vi "Periodic Tasks.vi"(8 "error in":errorcluster) -> ()   [LabVIEW 2020]
doc: "This VI runs in parallel to other tasks. It can contain as many user-defined periodic loops as you need. These can carry out PID or other sorts of timed response."
uses:
  <vilib>/Rock Robotics/WPI/ThirdParty/REV Robotics/REVLib/Typedef/Spark MAX Control Type.ctl
  <vilib>/Rock Robotics/WPI/Utilities/WPI_GetSetVariantRefNum.vi
panel:
  in  "Right Setpoint":dbl
  out "Right PID Chart":T1(graph)
  in  "Right PID Constants":T2={"P Gain"=0.0, "I Gain"=0.0, "D Gain"=0.0, "F Gain"=0.0, "I Zone"=0.0, "Min Output"=-1.0, "Max Output"=1.0} {"Max Output" min=-1.0 max=1.0 step=0.01; "Min Output" min=-1.0 max=1.0 step=0.01; "I Zone" step=0.01; "F Gain" step=0.01; "D Gain" step=0.01; "I Gain" step=0.01; "P Gain" min=0.0 step=0.01}
  in  "Left Setpoint":dbl
  out "Left PID Chart":T1(graph)
  in  "Left PID Constants":T2={"P Gain"=0.0, "I Gain"=0.0, "D Gain"=0.0, "F Gain"=0.0, "I Zone"=0.0, "Min Output"=-1.0, "Max Output"=1.0} {"Max Output" min=-1.0 max=1.0 step=0.01; "Min Output" min=-1.0 max=1.0 step=0.01; "I Zone" step=0.01; "F Gain" step=0.01; "D Gain" step=0.01; "I Gain" step=0.01; "P Gain" min=0.0 step=0.01}
  # "Click here to set max"
  # "Click here to set min"
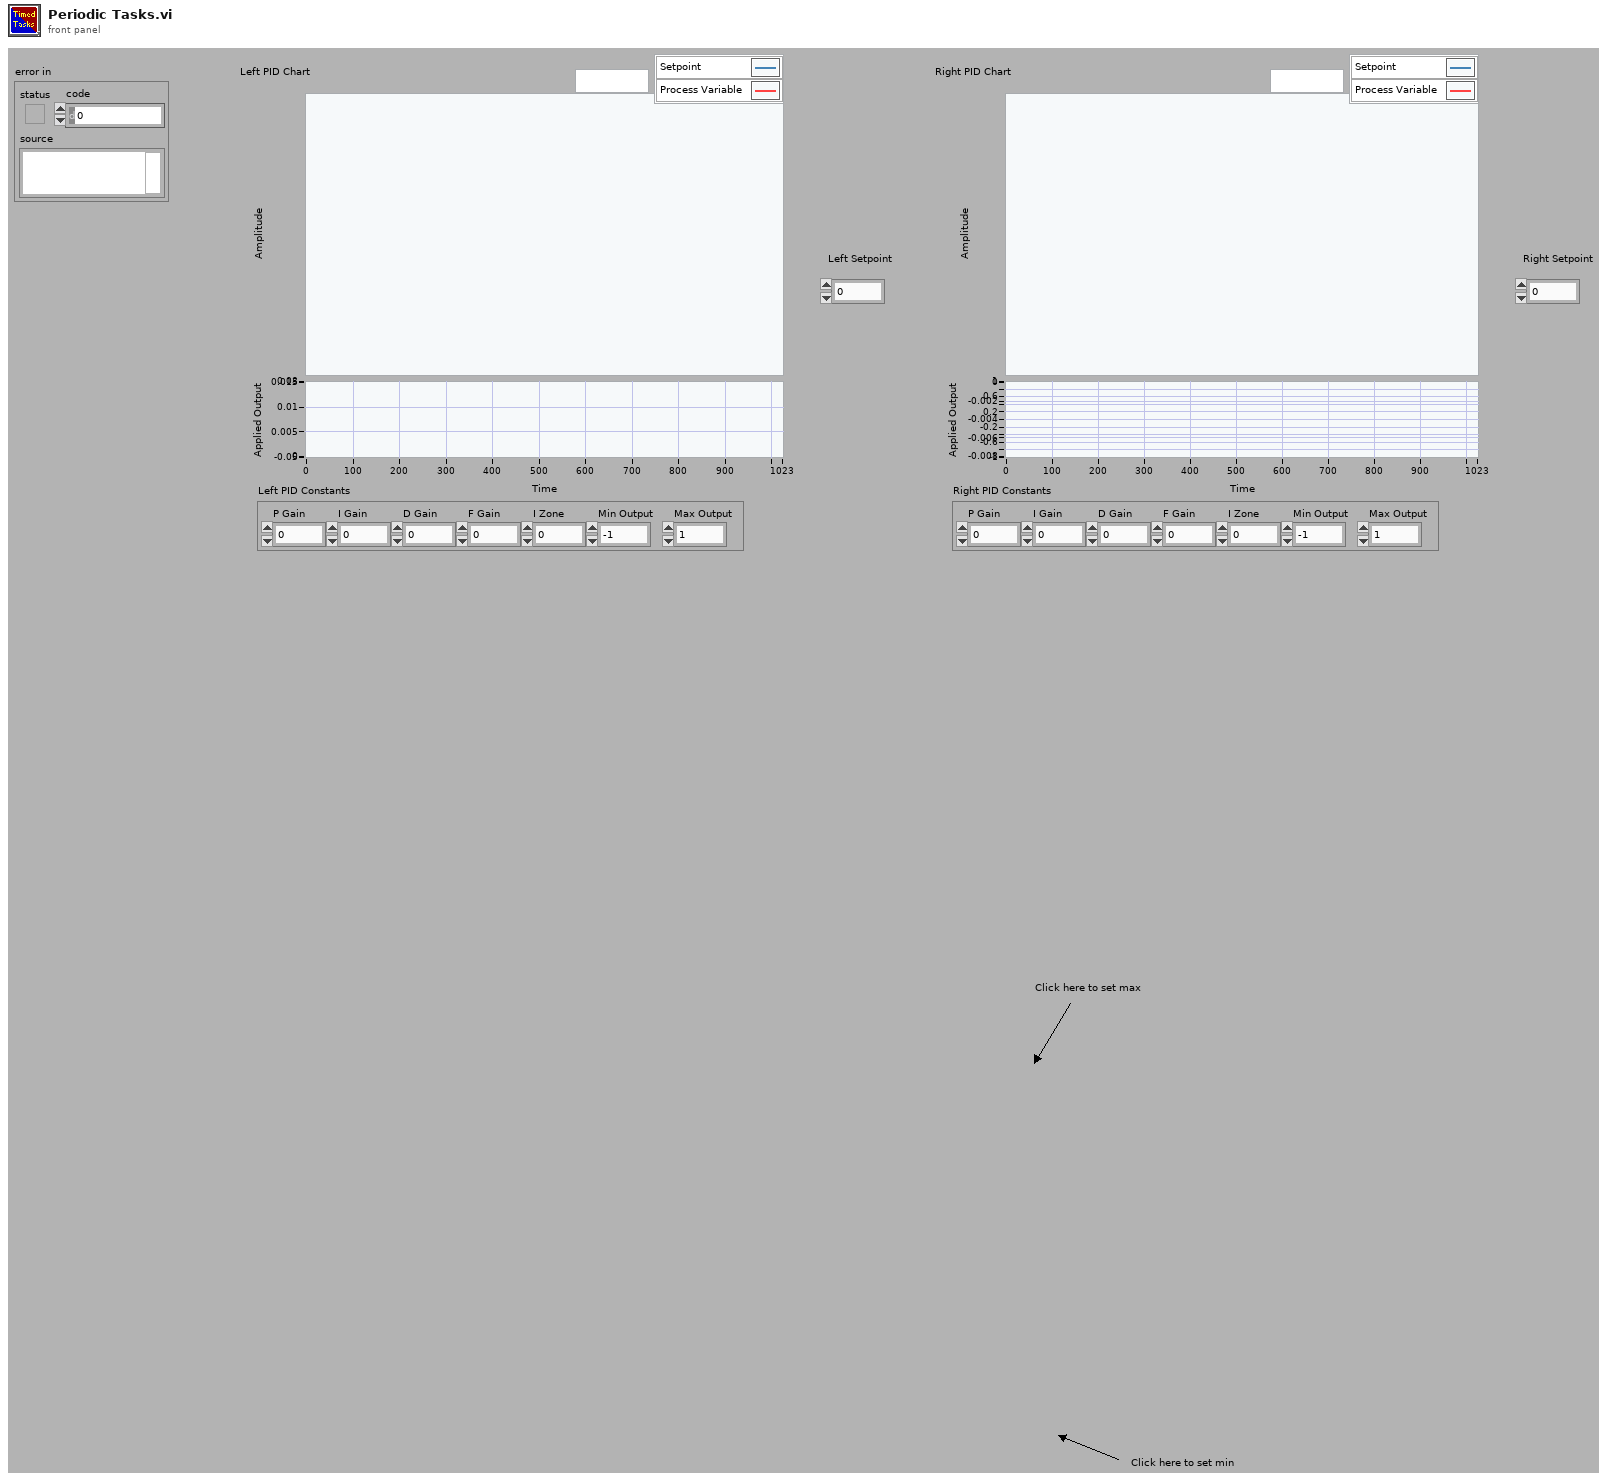
[diagram p1: front panel]
types:
  T1 = cluster{"Sensor Velocity":dbl, "Setpoint":dbl, "Applied Output":dbl}
  T2 = cluster{"P Gain":dbl, "I Gain":dbl, "D Gain":dbl, "F Gain":dbl, "I Zone":dbl, "Min Output":dbl, "Max Output":dbl}
  T3 = typedef "WPI_JoystickDevRef.ctl" = cluster{"Device":T4}
  T4 = typedef "WPI_JoystickDeviceEnum.ctl" = enum16{"USB 0", "USB 1", "USB 2", "USB 3", "USB 4", "USB 5"}
  T5 = typedef "WPI_RobotDriveDevRef.ctl" = cluster{"DevStatus":errorcluster, "Motors[]":T6[], "Square Inputs":bool, "Max Output":dbl}
  T6 = typedef "WPI_MotorControlDeviceRef.ctl" = cluster{"DeviceStatus":errorcluster, "Type":T7, "PWM":cluster{"PWM Channel":T8, "DeadBand":T9}, "CAN":cluster{"Device Number":u8, "SetOutput VI Ref":variant, "GetOutput VI Ref":variant, "Enable VI Ref":variant, "Disable VI Ref":variant, "Data":variant}, "Invert":bool, "DIO PWM":cluster{"PWM \"Enable\" Channel":T8, "DIOChannel":T10, "PWM Rate":dbl}}
  T7 = typedef "WPI_MotorControlType.ctl" = enum16{"PWM", "CAN", "DIO PWM"}
  T8 = typedef "FPGA_DIOPWMChannel.ctl" = enum8{"PWM 0", "PWM 1", "PWM 2", "PWM 3", "PWM 4", "PWM 5", "PWM 6", "PWM 7", "PWM 8", "PWM 9", "PWM MXP 0", "PWM MXP 1", "PWM MXP 2", "PWM MXP 3", "PWM MXP 4", "PWM MXP 5", "PWM MXP 6", "PWM MXP 7", "PWM MXP 8", "PWM MXP 9", "Invalid"}
  T9 = typedef "WPI_PWMDeadband.ctl" = cluster{"Name":string, "maxPositivePwm":i32, "minPositivePwm":i32, "centerPwm":i32, "maxNegativePwm":i32, "minNegativePwm":i32, "angularRange":u16}
  T10 = typedef "FPGA_DIOChannel.ctl" = enum8{"DIO 0", "DIO 1", "DIO 2", "DIO 3", "DIO 4", "DIO 5", "DIO 6", "DIO 7", "DIO 8", "DIO 9", "DIO MXP 0", "DIO MXP 1", "DIO MXP 2", "DIO MXP 3", "DIO MXP 4", "DIO MXP 5", "DIO MXP 6", "DIO MXP 7", "DIO MXP 8", "DIO MXP 9", "DIO MXP 10", "DIO MXP 11", "DIO MXP 12", "DIO MXP 13", "DIO MXP 14", "DIO MXP 15", "SPI Port CS1", "SPI Port CS2", "SPI Port CS3", "SPI Port MISO", "SPI Port MOSI", "Invalid"}
  T11 = cluster{"JoystickDevRef":T3, "RobotDriveDevRef":T5}
  T12 = typedef "Spark MAX Control Type.ctl" = enum16{"Percent VBus", "Voltage", "Velocity", "Position", "Smart Motion", "Current", "Smart Velocity"}
  T13 = cluster{"P Gain":bool, "I Gain":bool, "D Gain":bool, "F Gain":bool, "I Zone":bool, "Min Output":bool, "Max Output":bool}
  T14 = typedef "Spark MAX Status 2 Frame.ctl" = cluster{"Sensor Position":dbl, "IAccum":dbl, "Timestamp":u32}
  T15 = typedef "Spark MAX Status 0 Frame.ctl" = cluster{"Applied Output":dbl, "Faults":T16, "Sticky Faults":T16, "Rsvd":u8, "Status 0 Flags":T17, "Timestamp":u32}
  T16 = typedef "Spark MAX Faults.ctl" = cluster{"Hard Limit Rev":bool, "Hard Limit Fwd":bool, "Soft Limit Fwd":bool, "Soft Limit Rev":bool, "Other Fault":bool, "DRV Fault":bool, "Has Reset?":bool, "CAN RX":bool, "CAN TX":bool, "EEPROM CRC":bool, "Stall":bool, "Sensor Fault":bool, "Motor Type Fault":bool, "IWDT Reset":bool, "Over Current":bool, "Brownout":bool}
  T17 = typedef "Spark MAX Status 0 Flags.ctl" = cluster{"Invert/Brake":bool, "Is Follower":bool}
  T18 = cluster{"Sensor Position":dbl, "Right Setpoint":dbl, "Applied Output":dbl}
  T19 = cluster{"Sensor Position":dbl, "Left Setpoint":dbl, "Applied Output":dbl}
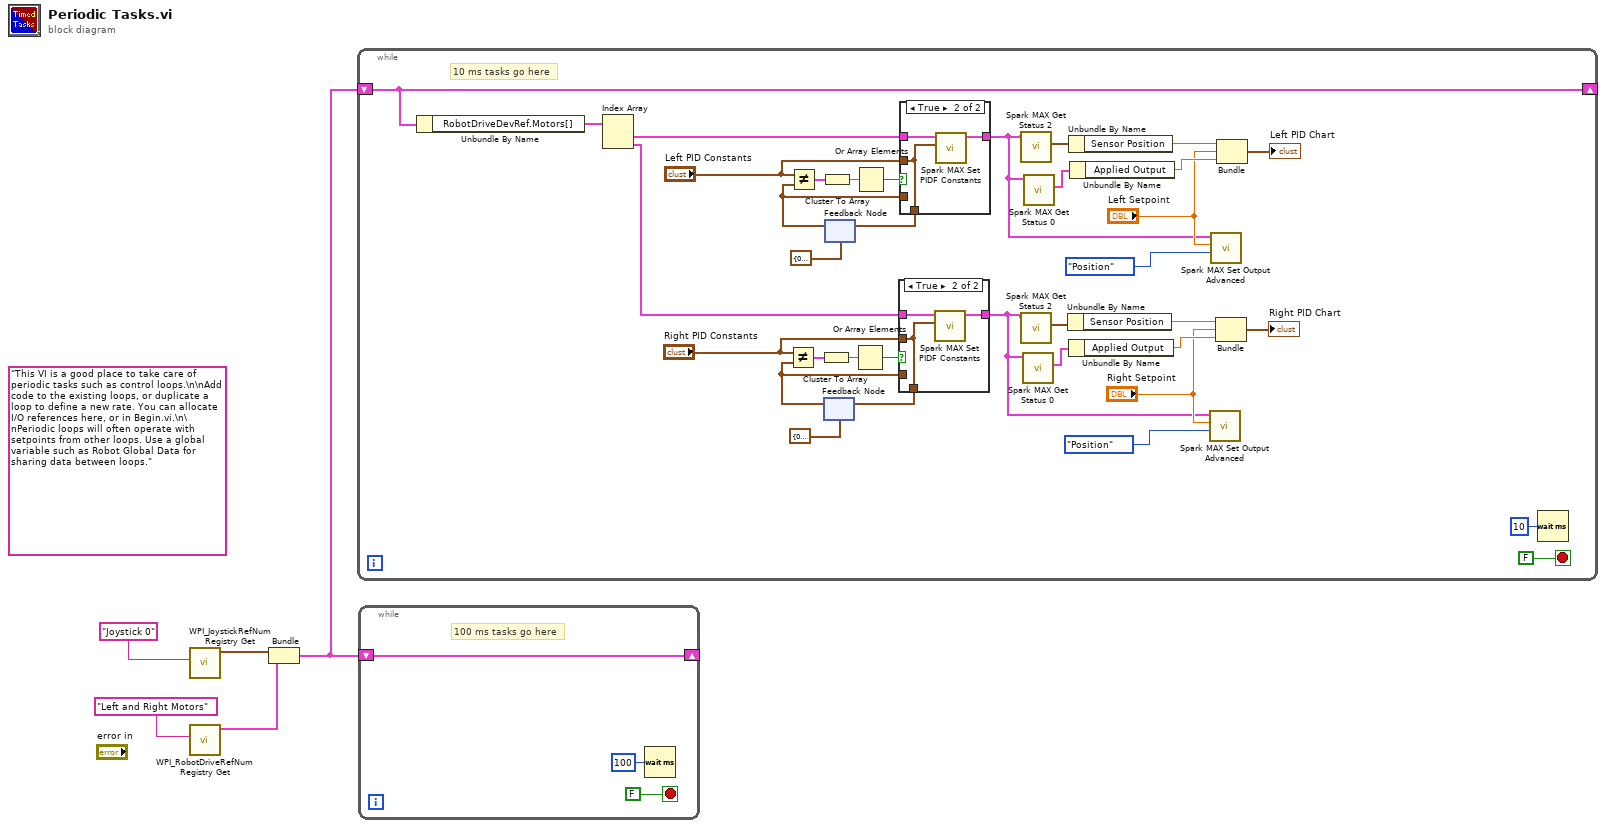
[diagram p0: block diagram]
diagram:
  (unwired) "This VI is a good place to take care of periodic tasks such as control loops.\n\nAdd code to the existing loops, or duplicate a loop to define a new rate. You can allocate I/O references here, or in Begin.vi.\n\nPeriodic loops will often operate with setpoints from other loops. Use a global variable such as Robot Global Data for sharing data between loops."
  n1 = call <vilib>:"WPI_JoystickRefNum Registry Get.vi"("refnum name"="Joystick 0") -> ("JoystickDevRef"=w3:T3)  [unwired: 1 in, 9 out]
  n2 = call <vilib>:"WPI_RobotDriveRefNum Registry Get.vi"("refnum name"="Left and Right Motors") -> ("RobotDriveDevRef"=w2:T5)  [unwired: 1 in, 9 out]
  n3 = Bundle("JoystickDevRef"=w3, "RobotDriveDevRef"=w2) -> (w1:T11)  [unwired: 1 out]
  n4 = while {
    shift-right: [w10] -> _
    shift-left: w1 -> [w10]
    stop <- FALSE stop-if-true
    # "10 ms tasks go here"
    n5 = Unbundle By Name(w10) -> ("RobotDriveDevRef.Motors[]"=w26:T6[])
    n6 = Index Array(array=w26) -> (element #1=w25:T6, element #2=w11:T6)  [unwired: 2 in]
    n7 = feedback #1(T2 {"P Gain"=0.0, "I Gain"=0.0, "D Gain"=0.0, "F Gain"=0.0, "I Zone"=0.0, "Min Output"=0.0, "Max Output"=0.0} ("PID Constants")) -> (w18:T2)
    n8 = Not Equal?(x="Right PID Constants", y=w18) -> (x != y?=w12:T13)
    n9 = Cluster To Array(cluster=w12) -> (array=w13:bool[])
    n10 = feedback #2(T2 {"P Gain"=0.0, "I Gain"=0.0, "D Gain"=0.0, "F Gain"=0.0, "I Zone"=0.0, "Min Output"=0.0, "Max Output"=0.0} ("PID Constants")) -> (w33:T2)
    n11 = Not Equal?(x="Left PID Constants", y=w33) -> (x != y?=w27:T13)
    n12 = Cluster To Array(cluster=w27) -> (array=w28:bool[])
    n13 = Or Array Elements(Boolean array=w13) -> (logical OR=w15:bool)
    n14 = Or Array Elements(Boolean array=w28) -> (logical OR=w30:bool)
    n15 = case shown="True" w15 {
      tunnel: w11 -> [w42 w46]
      tunnel: "Right PID Constants" -> [_ w44]
      tunnel: [w43 w44] -> w17
      tunnel: w18 -> [w43 _]
      tunnel: [w42 w45] -> w7
      frame False {
      }
      frame True {
        n16 = call <vilib>:"Spark MAX Set PIDF Constants.vi"("PID Constants"=w44, "MotorControlDeviceRef"=w46) -> ("MotorControlDeviceRef"=w45:T6)  [unwired: 8 in, 1 out]
      }
    }
    n17 = feedback-in #1(w17) -> ()
    n18 = case shown="True" w30 {
      tunnel: w25 -> [w47 w51]
      tunnel: "Left PID Constants" -> [_ w49]
      tunnel: [w48 w49] -> w32
      tunnel: w33 -> [w48 _]
      tunnel: [w47 w50] -> w9
      frame False {
      }
      frame True {
        n19 = call <vilib>:"Spark MAX Set PIDF Constants.vi"("PID Constants"=w49, "MotorControlDeviceRef"=w51) -> ("MotorControlDeviceRef"=w50:T6)  [unwired: 8 in, 1 out]
      }
    }
    n20 = feedback-in #2(w32) -> ()
    n21 = call <vilib>:"Spark MAX Get Status 2.vi"("MotorControlDevRef"=w9) -> ("Stat 2"=w8:T14)  [unwired: 7 in, 3 out]
    n22 = call <vilib>:"Spark MAX Get Status 2.vi"("MotorControlDevRef"=w7) -> ("Stat 2"=w6:T14)  [unwired: 7 in, 3 out]
    n23 = call <vilib>:"Spark MAX Get Status 0.vi"("MotorControlDevRef"=w7) -> ("Status 0"=w23:T15)  [unwired: 7 in, 3 out]
    n24 = call <vilib>:"Spark MAX Get Status 0.vi"("MotorControlDevRef"=w9) -> ("Status 0"=w38:T15)  [unwired: 7 in, 3 out]
    n25 = Unbundle By Name(w6) -> ("Sensor Position"=w19:dbl)
    n26 = Unbundle By Name(w8) -> ("Sensor Position"=w34:dbl)
    n27 = Unbundle By Name(w23) -> ("Applied Output"=w24:dbl)
    n28 = Unbundle By Name(w38) -> ("Applied Output"=w39:dbl)
    n29 = call <vilib>:"Spark MAX Set Output Advanced.vi"("Control Mode"=Spark_MAX_Control_Type."Position", "Setpoint"="Right Setpoint", "MotorControlDevRef"=w7) -> ()  [unwired: 7 in, 2 out]
    n30 = call <vilib>:"Spark MAX Set Output Advanced.vi"("Control Mode"=Spark_MAX_Control_Type."Position", "Setpoint"="Left Setpoint", "MotorControlDevRef"=w9) -> ()  [unwired: 7 in, 2 out]
    n31 = Bundle("Sensor Position"=w19, "Right Setpoint"="Right Setpoint", "Applied Output"=w24) -> (→"Right PID Chart":T18)  [unwired: 1 in]
    n32 = Bundle("Sensor Position"=w34, "Left Setpoint"="Left Setpoint", "Applied Output"=w39) -> (→"Left PID Chart":T19)  [unwired: 1 in]
    n33 = Wait (ms)(milliseconds to wait=u32 10) -> ()  [unwired: 1 out]
  }
  n34 = while {
    shift-right: [w52] -> _
    shift-left: w1 -> [w52]
    stop <- FALSE stop-if-true
    # "100 ms tasks go here"
    n35 = Wait (ms)(milliseconds to wait=u32 100) -> ()  [unwired: 1 out]
  }
